vi "OCV Get Frame to Array.vi"(8 "error in (no error)":errorcluster) -> (0 "error out":errorcluster, 3 "frame":u32[][](array[numeric]))   [LabVIEW 2018, in "OpenCVcamLV.lvlib"]
uses:
  OpenCVcamLV.lvlib
  LVopenCVcamDLL.dll
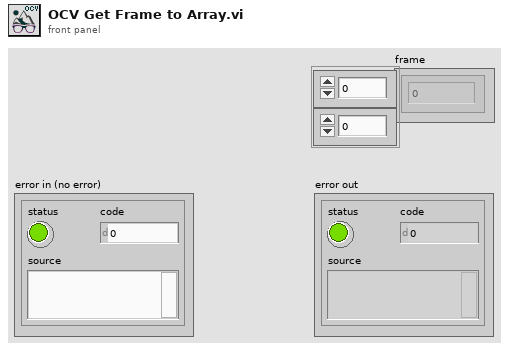
[diagram p1: front panel]
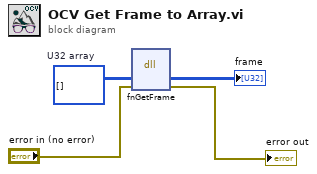
[diagram p0: block diagram]
diagram:
  w2 = u32[][] []  # U32 array
  n1 = dll-call lib="C:/Users/Andrey/Desktop/OpenCVcamLV/LVopenCVcamDLL.dll" fn="fnGetFrame"("frame"=w2, "err"="error in (no error)") -> ("frame"=→"frame":u32[][], "err"=→"error out":errorcluster)  [unwired: 4 in, 2 out]
